vi "CTRE_CANTalonSRX_GetVelocityMeasurementPeriod.vi"(8 "error in (no error)":errorcluster, 11 "CAN Talon SRX Ref":T1={"DeviceStatus"={"status"=FALSE, "code"=0, "source"=""}, "Type"=enum."PWM", "PWM"={"PWM Channel"=enum."PWM 1", "DeadBand"={"Name"="", "maxPositivePwm"=0, "minPositivePwm"=0, "centerPwm"=0, "maxNegativePwm"=0, "minNegativePwm"=0, "angularRange"=0}}, "CAN"={"Device Number"=0, "SetOutput VI Ref"=variant(enum8{"Percent VBus", "Current", "Speed", "Position", "Voltage"} enum."Percent VBus"), "GetOutput VI Ref"=variant(refnum<k1> refnum), "Enable VI Ref"=variant(dbl 12.0), "Disable VI Ref"=variant(enum8{"Percent VBus", "Speed", "Position", "Slave", "Unchanged / Invalid", "Voltage Compensation", "Current", "Motion Profile"} enum."Percent VBus"), "Data"=variant}, "Invert"=FALSE}) -> (0 "error out":errorcluster, 2 "Velocity Measurement Period":dbl, 3 "CAN Talon SRX Ref":T1={"DeviceStatus"={"status"=FALSE, "code"=0, "source"=""}, "Type"=enum."PWM", "PWM"={"PWM Channel"=enum."Invalid", "DeadBand"={"Name"="", "maxPositivePwm"=0, "minPositivePwm"=0, "centerPwm"=0, "maxNegativePwm"=0, "minNegativePwm"=0, "angularRange"=0}}, "CAN"={"Device Number"=0, "SetOutput VI Ref"=variant, "GetOutput VI Ref"=variant, "Enable VI Ref"=variant, "Disable VI Ref"=variant, "Data"=variant}, "Invert"=FALSE})   [LabVIEW 2016]
uses:
  <vilib>/Rock Robotics/WPI/MotorControl/WPI_MotorControlDeviceRef.ctl
  <vilib>/Rock Robotics/WPI/MotorControl/WPI_MotorControlType.ctl
  <vilib>/Rock Robotics/SystemInterfaces/DIO/FPGA_DIOPWMChannel.ctl
  <vilib>/Rock Robotics/WPI/PWM/WPI_PWMDeadband.ctl
  <vilib>/Rock Robotics/WPI/ThirdParty/CanMotor/TalonSRX/WPI_CANTalonSRX_Params.ctl
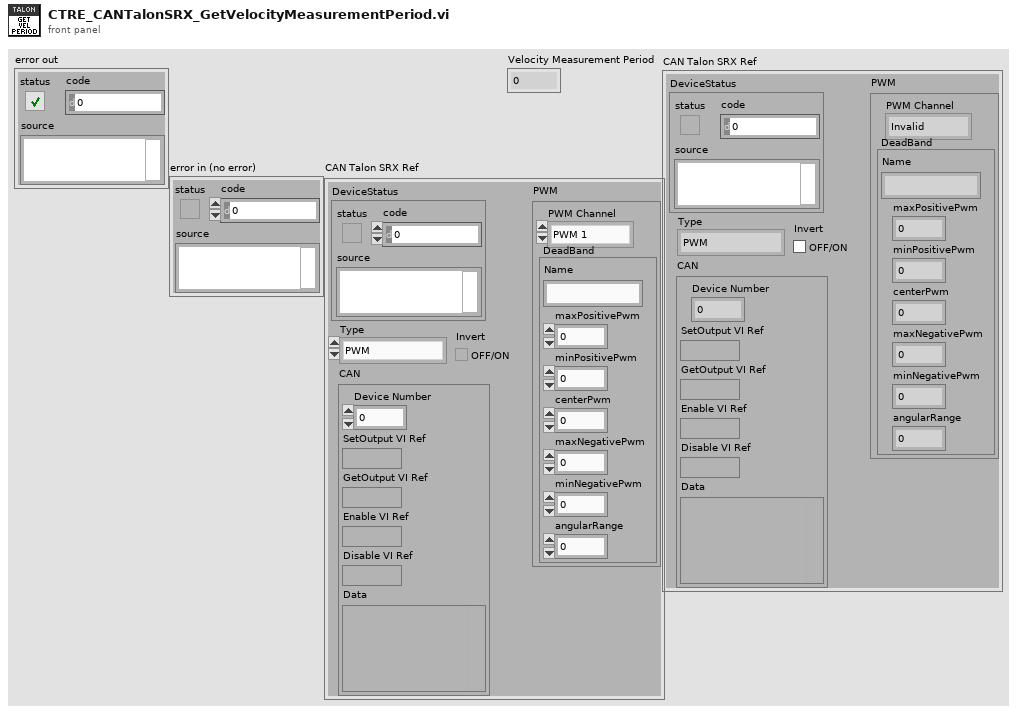
[diagram p1: front panel]
types:
  T1 = typedef "WPI_MotorControlDeviceRef.ctl" = cluster{"DeviceStatus":errorcluster, "Type":T2, "PWM":cluster{"PWM Channel":T3, "DeadBand":T4}, "CAN":cluster{"Device Number":u8, "SetOutput VI Ref":variant, "GetOutput VI Ref":variant, "Enable VI Ref":variant, "Disable VI Ref":variant, "Data":variant}, "Invert":bool}
  T2 = typedef "WPI_MotorControlType.ctl" = enum16{"PWM", "CAN"}
  T3 = typedef "FPGA_DIOPWMChannel.ctl" = enum8{"PWM 0", "PWM 1", "PWM 2", "PWM 3", "PWM 4", "PWM 5", "PWM 6", "PWM 7", "PWM 8", "PWM 9", "PWM MXP 0", "PWM MXP 1", "PWM MXP 2", "PWM MXP 3", "PWM MXP 4", "PWM MXP 5", "PWM MXP 6", "PWM MXP 7", "PWM MXP 8", "PWM MXP 9", "Invalid"}
  T4 = typedef "WPI_PWMDeadband.ctl" = cluster{"Name":string, "maxPositivePwm":i32, "minPositivePwm":i32, "centerPwm":i32, "maxNegativePwm":i32, "minNegativePwm":i32, "angularRange":u16}
  T5 = typedef "WPI_CANTalonSRX_Params.ctl" = u8
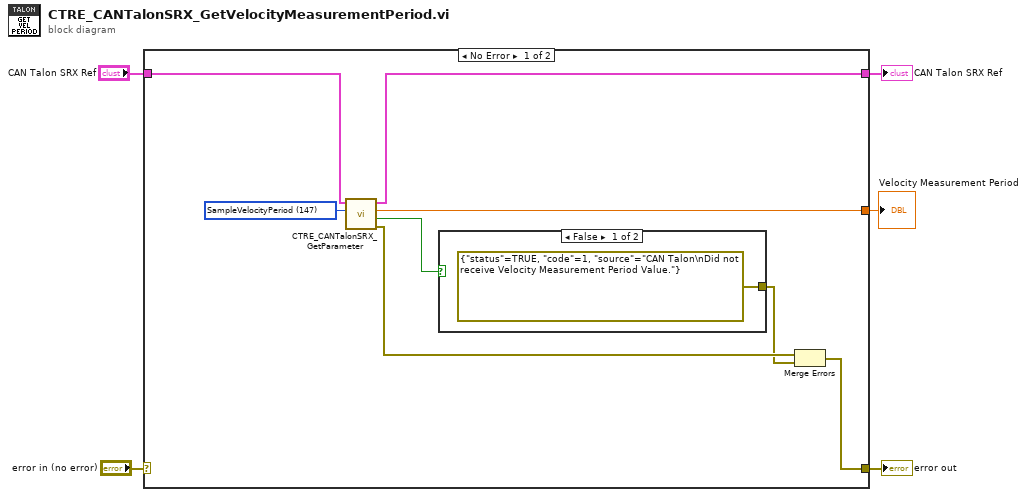
[diagram p0: block diagram]
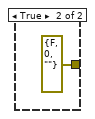
[diagram p2: hidden frame]
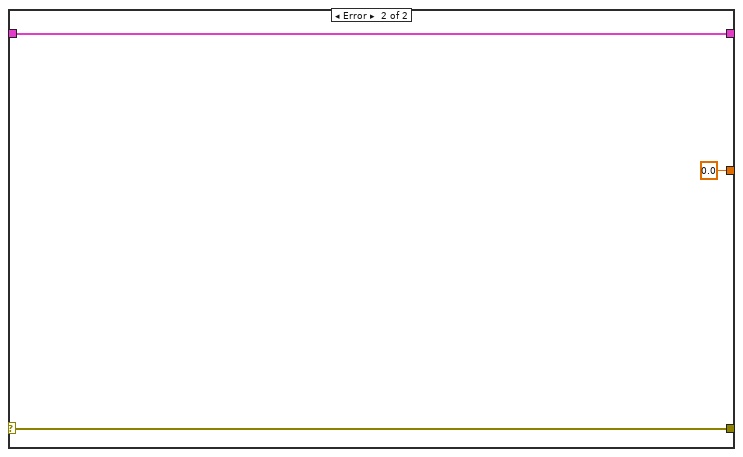
[diagram p3: hidden frame]
diagram:
  n1 = case shown="No Error" "error in (no error)" {
    selector: "error in (no error)" -> [_ w18]
    tunnel: "CAN Talon SRX Ref" -> [w12 w17]
    tunnel: [w11 0.0 ("Parameter Value")] -> w3
    tunnel: [w10 w17] -> w2
    tunnel: [w6 w18] -> w1
    frame No Error {
      w13 = T5 147 items=["Slot 0 - P"=1, "Slot 0 - I"=2, "Slot 0 - D"=3, "Slot 0 - F"=4, "Slot 0 - I Zone"=5, "Slot 0 - Ramp Rate"=6, "Slot 1 - P"=11, "Slot 1 - I"=12, "Slot 1 - D"=13, "Slot 1 - F"=14, "Slot 1 - I Zone"=15, "Slot 1 - Ramp Rate"=16, "Soft Limit - Forward"=21, "Soft Limit - Reverse"=22, "Soft Limit - Forward Enable"=23, "Soft Limit - Reverse Enable"=24, "On Boot - Brake Mode"=31, "On Boot - Limit Normally Closed - Forward"=32, "On Boot - Limit Normally Closed - Reverse"=33, "On Boot - Limit Disabled - Forward"=34, "On Boot - Limit Disabled - Reverse"=35, "Fault - Over Temp"=41, "Fault - Under Voltage"=42, "Fault - Forward Limit"=43, "Fault - Reverse Limit"=44, "Fault - Hardware Failure"=45, "Fault - Forward Soft Limit"=46, "Fault - Reverse Soft Limit"=47, "Sticky Fault - Over Temp"=48, "Sticky Fault - Under Voltage"=49, "Sticky Fault - Forward Limit"=50, "Sticky Fault - Reverse Limit"=51, "Sticky Fault - Forward Soft Limit"=52, "Sticky Fault - Reverse Soft Limit"=53, "Applied Throttle"=61, "Closed-Loop Error"=62, "Select Feedback Device"=63, "Reverse Closed-Loop Output"=64, "Mode Select"=65, "Profile Slot Select"=66, "Ramp Throttle"=67, "Reverse Feedback Sensor"=68, "Limit Switch Enabled"=69, "Limit Switch Closed - Forward"=70, "Limit Switch Closed - Reverse"=71, "Sensor Position"=73, "Sensor Velocity"=74, "Current"=75, "Brake is Enabled"=76, "Encoder Position"=77, "Encoder Velocity"=78, "Encoder Index Rise Events"=79, "Encoder A Pin State"=80, "Encoder B Pin State"=81, "Encoder Index Pin State"=82, "Analog In with Overflow"=83, "Analog In Velocity"=84, "Temperature"=85, "Battery Voltage"=86, "Reset Count"=87, "Reset Flags"=88, "Firmware Version"=89, "Settings Changed"=90, "Quad Filter Enable"=91, "Ignore Disable Broadcast"=92, "I Accumulator"=93, "Status 1 Frame Rate Ms"=94, "Status 2 Frame Rate Ms"=95, "Status 3 Frame Rate Ms"=96, "Status 4 Frame Rate Ms"=97, "Status 6 Frame Rate Ms"=98, "Status 7 Frame Rate Ms"=99, "Enable Index Pin Clear Position"=100, "Peak Positive Output"=104, "Nominal Positive Output"=105, "Peak Negative Output"=106, "Nominal Negative Output"=107, "Quad Index Pin Polarity"=108, "Status 8 Frame Rate Ms"=109, "Allow Position Overflow"=110, "Slot 0 - Allowable Closed-Loop Error"=111, "Number Potentiometer Turns"=112, "Encoder Codes Per Rev"=113, "Pulse Width Decoded Position"=114, "Analog Position"=115, "Voltage Compensation Rate (V/s)"=116, "Slot 1 - Allowable Closed-Loop Error"=117, "Motion Profile Has Underrun Err"=119, "Reserved 120"=120, "Legacy Control Mode"=121, "Motion Magic Acceleration"=122, "Motion Magic Cruise Velocity"=123, "Status 10 Frame Rate"=124, "Current Limit Threshold"=125, "CustomParam0"=137, "CustomParam1"=138, "PersStorageSaving"=139, "ClearPositionOnLimitF"=144, "ClearPositionOnLimitR"=145, "NominalBatteryVoltage"=146, "SampleVelocityPeriod"=147, "SampleVelocityWindow"=148] ("Parameter")
      n2 = call <vilib>:"CTRE_CANTalonSRX_GetParameter.vi"("Parameter"=w13, "CAN Talon SRX Ref"=w12) -> ("error out"=w8:errorcluster, "Value Received?"=w9:bool, "Parameter Value"=w11:dbl, "CAN Talon SRX Ref"=w10:T1)  [unwired: 6 in]
      n3 = case shown="False" w9 {
        tunnel: [errorcluster {"status"=TRUE, "code"=1, "source"="CAN Talon\nDid not receive Velocity Measurement Period Value."} ("error out") errorcluster {"status"=FALSE, "code"=0, "source"=""} ("error out")] -> w7
        frame False {
        }
        frame True {
        }
      }
      n4 = Merge Errors(w8, w7) -> (w6:errorcluster)
    }
    frame Error {
    }
  }
  "Velocity Measurement Period" <- w3
  "CAN Talon SRX Ref" <- w2
  "error out" <- w1
